vi "Handle Last Ack Core.vi"(4 "error in (no error)":errorcluster, 6 "Last Ack":refnum<class "Last Ack.lvclass">, 7 "Vehicle Position Interface Simulation in":refnum<class "Vehicle Position Interface Simulation.lvclass">) -> (0 "error out":errorcluster, 3 "Vehicle Position Interface Simulation out":refnum<class "Vehicle Position Interface Simulation.lvclass">)   [LabVIEW 2012, in "Vehical Position Interface Simulation.lvlib" / "Vehicle Position Interface Simulation.lvclass"]
doc: "(<B>Filename</B>: Actor Framework.lvlib:Actor.lvclass:Handle Last Ack Core.vi)\n\nDefines how the caller actor responds to the Last Ack message from a nested actor. The Last Ack message is the final message a nested actor sends to its caller before it shuts down. The message contains information about the final state of the nested actor.\n\nBy default, this method does nothing except return any error the nested actor sent. A descendant class may override this method to define behavior."
uses:
  Vehicle Position Interface Simulation.lvclass
  Vehical Position Interface API/Vehical Position Interface API/Vehicle Position Interface API.lvclass
  <vilib>/ActorFramework/LastAck/Last Ack.lvclass
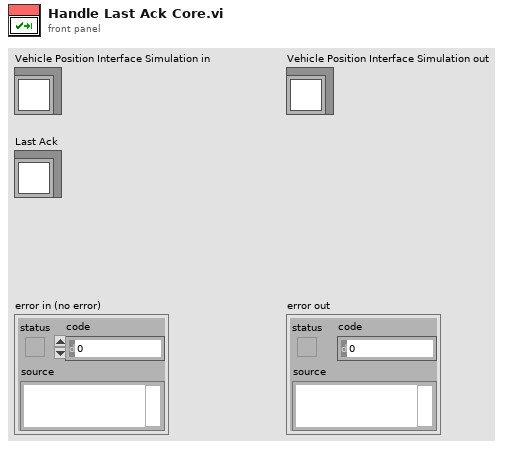
[diagram p1: front panel]
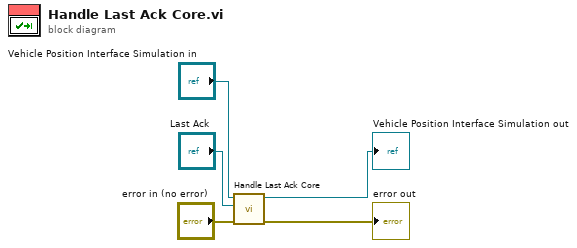
[diagram p0: block diagram]
diagram:
  n1 = call-parent "Handle Last Ack Core.vi"("error in (no error)"="error in (no error)", "Last Ack"="Last Ack", "Actor in"="Vehicle Position Interface Simulation in") -> ("error out"=→"error out":errorcluster, "Actor out"=→"Vehicle Position Interface Simulation out":refnum<class "Vehicle Position Interface Simulation.lvclass">)  [unwired: 3 in]
